vi "Intensity_png.vi"(3 "No of Contours":i32=20, 4 "Job Directory":path=path "/Lacie_20/paulhayden/Documents/EnFlo bits/EnFlo Tun Vel profiles/View_LDA data.tpt", 5 "Intensity Graph":dbl[][](graph)) -> ()   [LabVIEW 2015]
uses:
  Results_plotter_Global.vi
panel:
  out "Folders":string[](array[string])
  out "String":string
  in  "Added labels":i32[](listbox)
  in  "Z Min":dbl=0.97
  in  "Z Max":dbl=1.07
  in  "Save Automatically?":bool
  in  "Auto scale Intensity":bool=TRUE
  in  "Colour":bool=TRUE
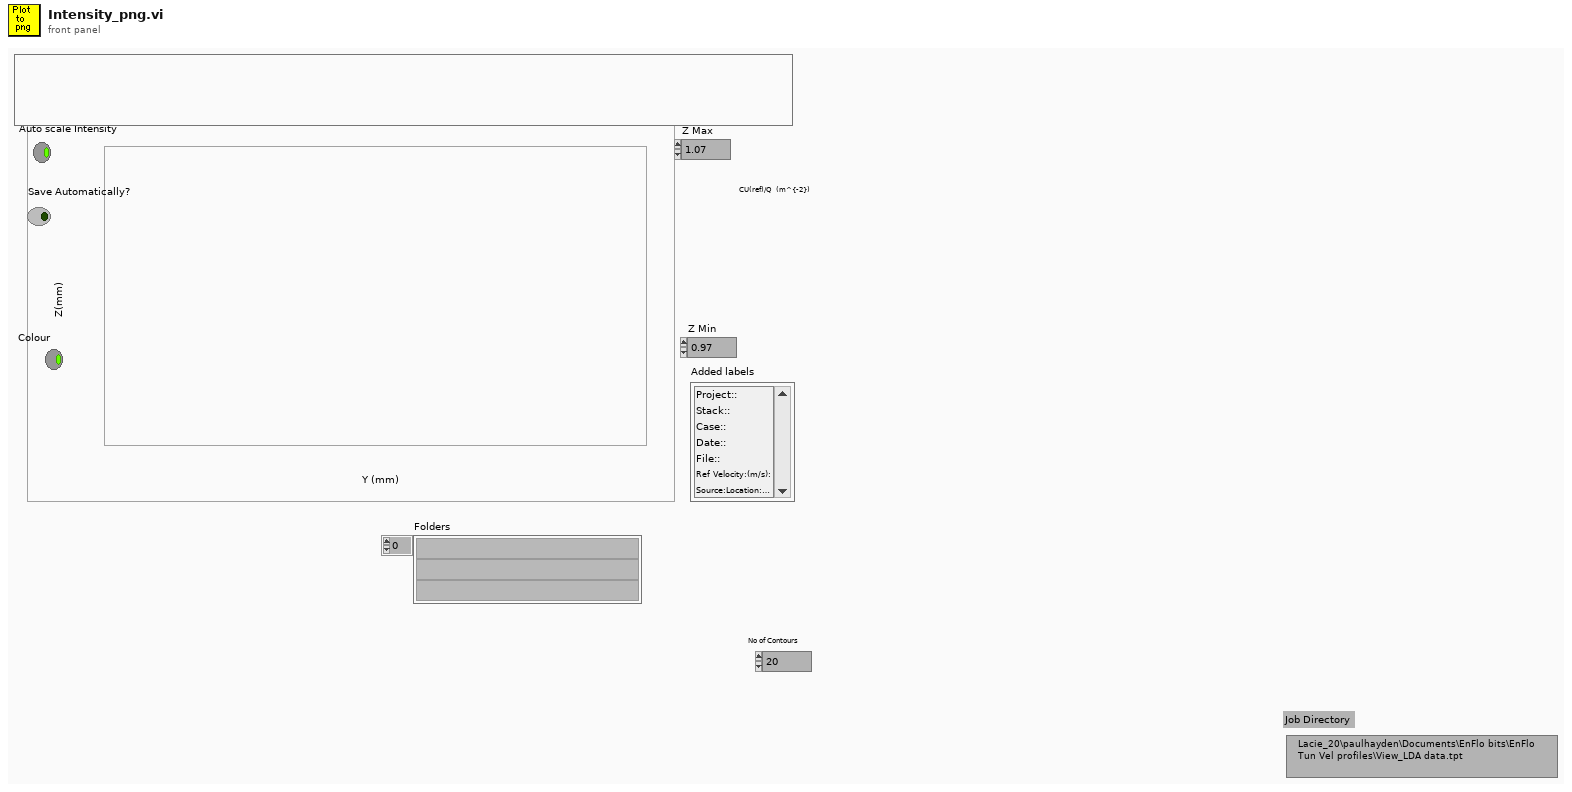
[diagram p1: front panel]
types:
  T1 = typedef "LVRectTypeDef.ctl" = cluster{"left":i16, "top":i16, "right":i16, "bottom":i16}
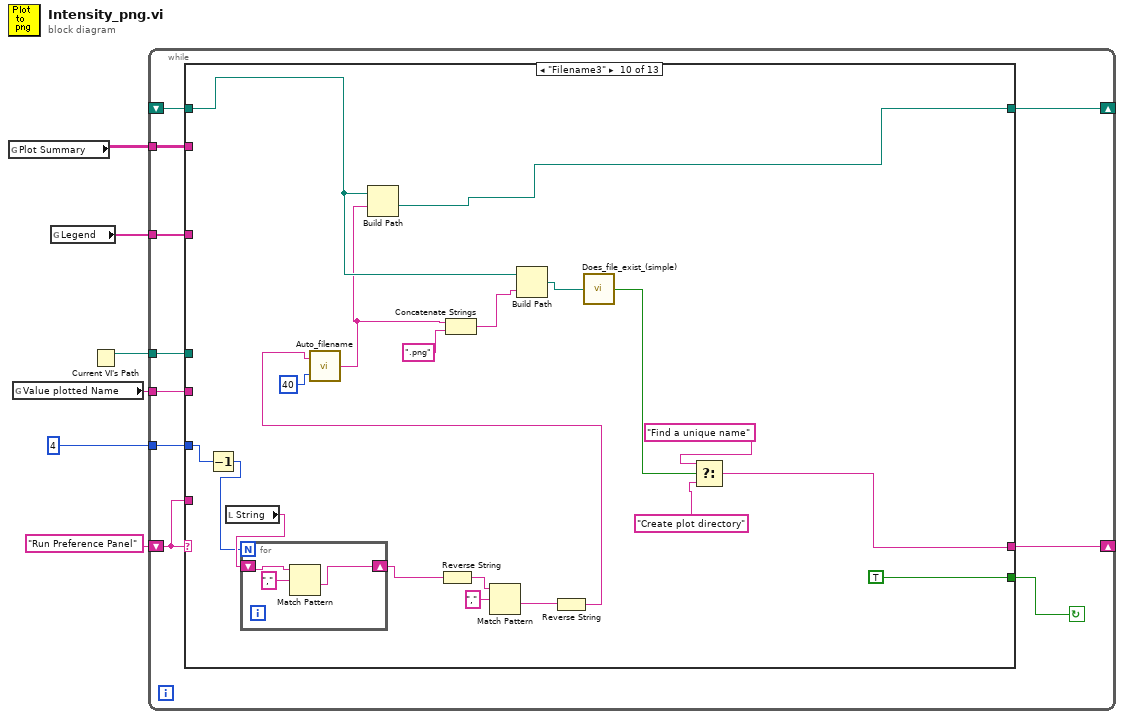
[diagram p0: block diagram]
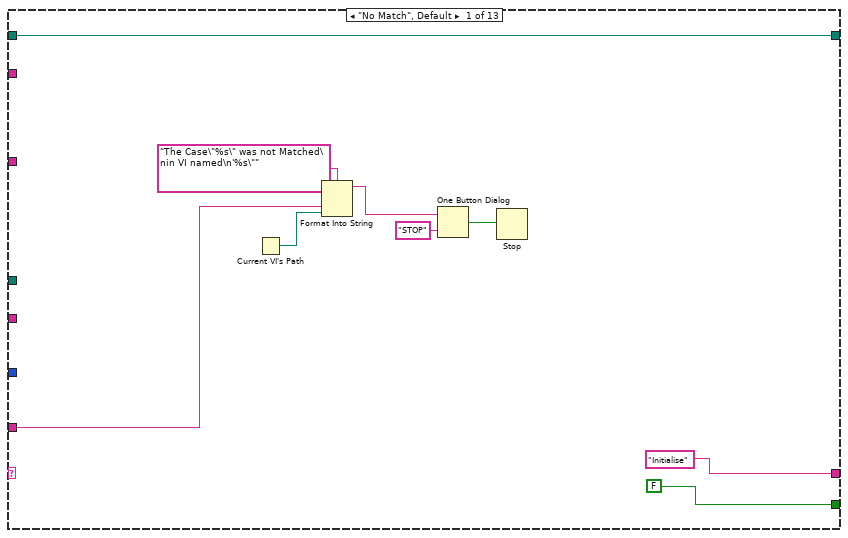
[diagram p2: hidden frame]
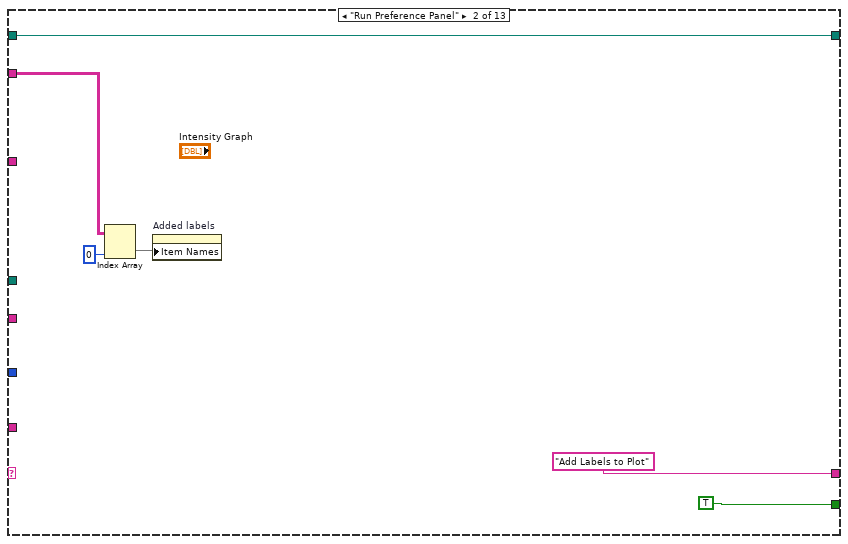
[diagram p3: hidden frame]
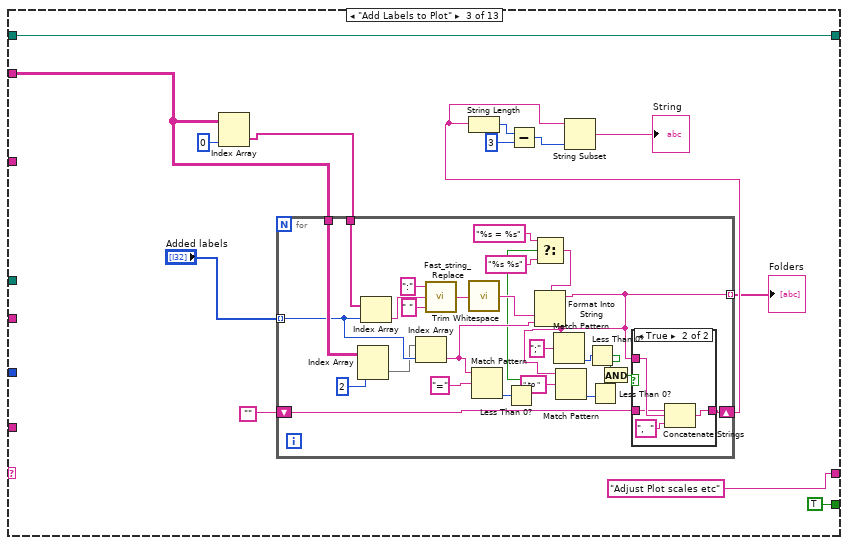
[diagram p4: hidden frame]
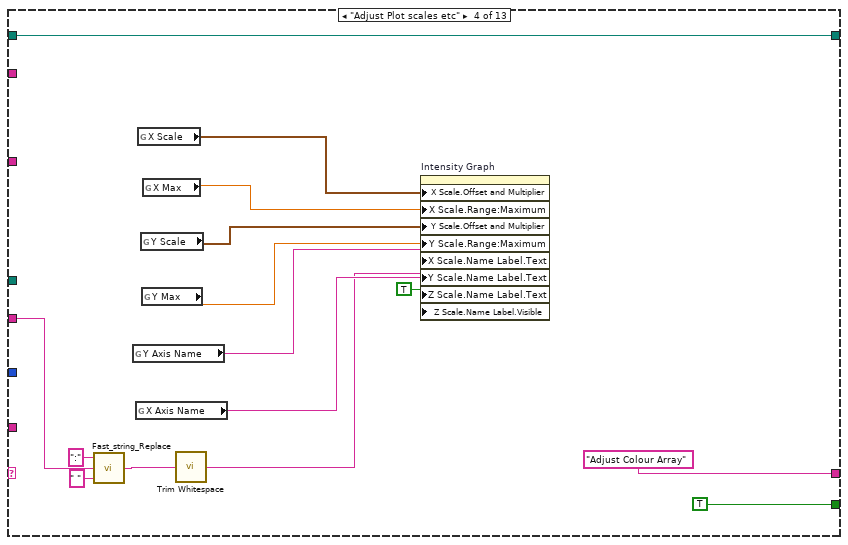
[diagram p6: hidden frame]
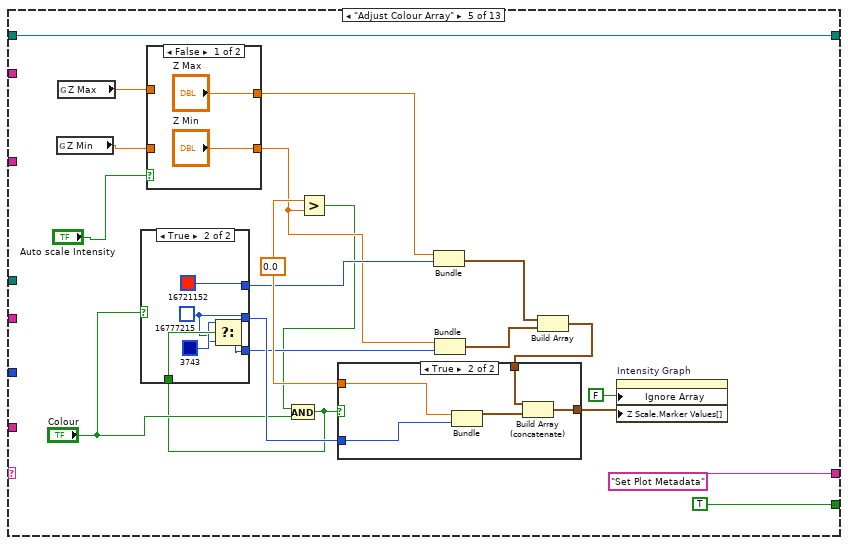
[diagram p7: hidden frame]
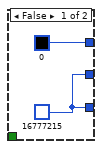
[diagram p8: hidden frame]
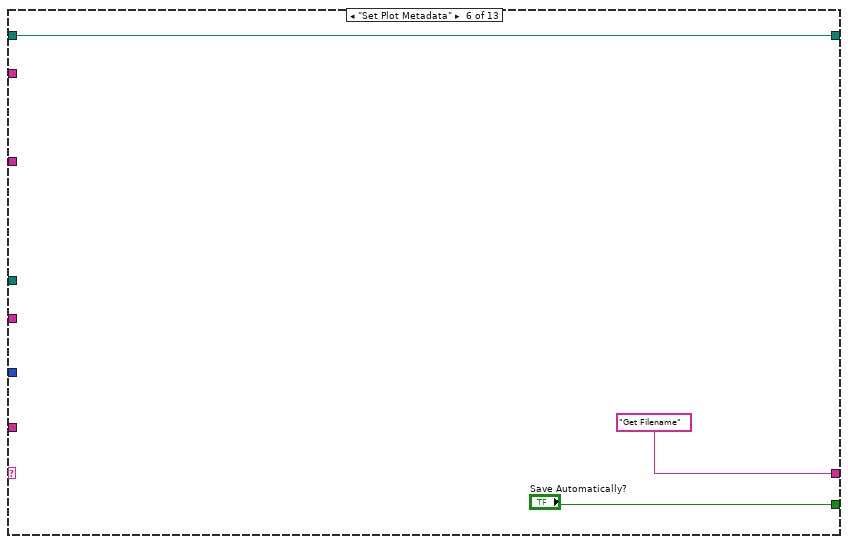
[diagram p11: hidden frame]
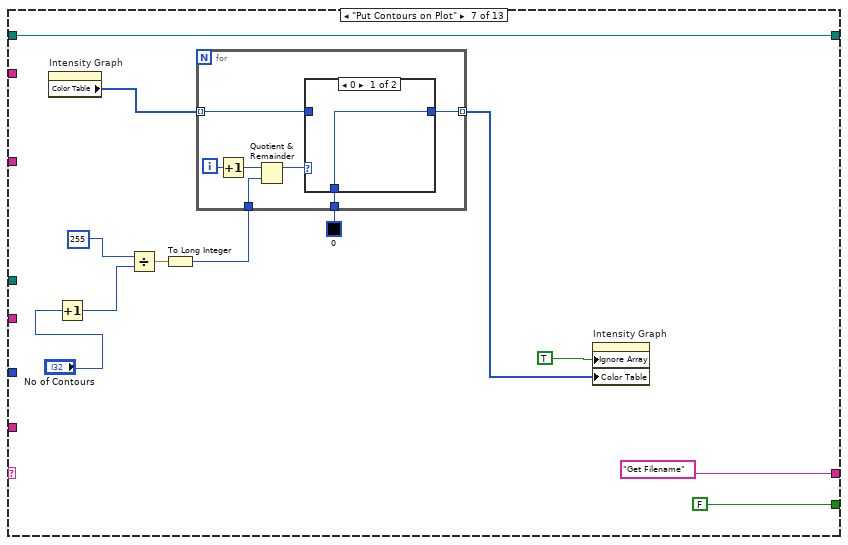
[diagram p12: hidden frame]
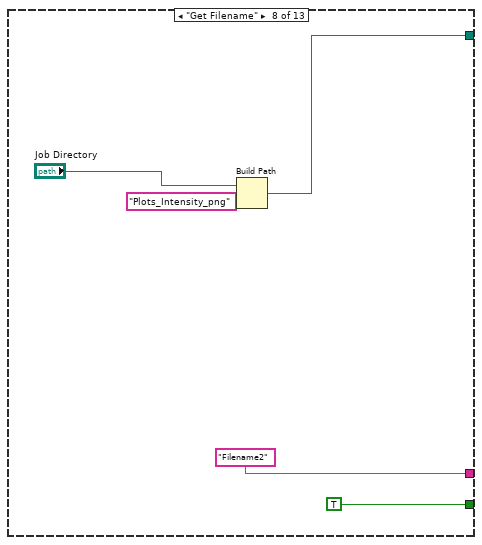
[diagram p14: hidden frame]
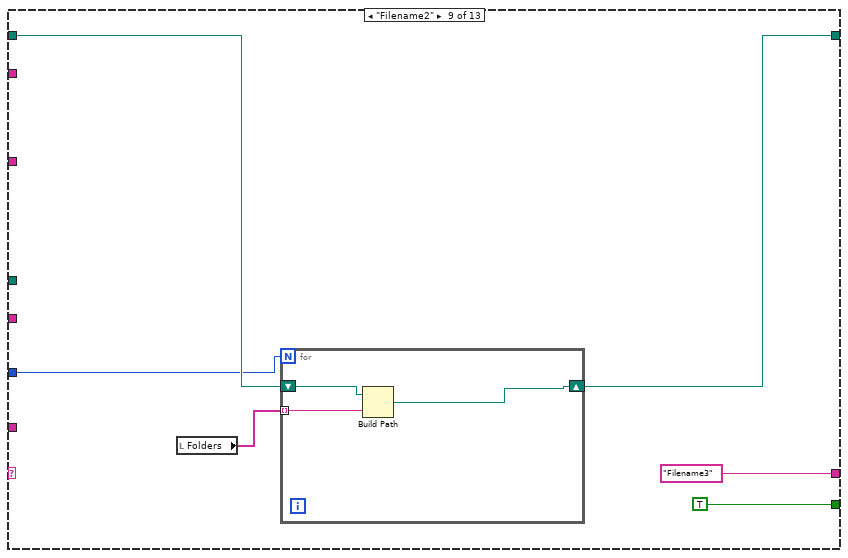
[diagram p15: hidden frame]
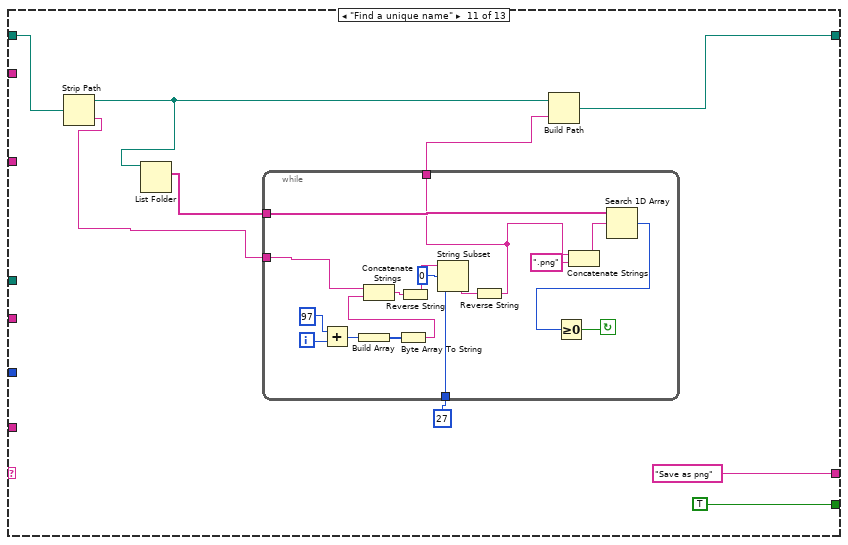
[diagram p16: hidden frame]
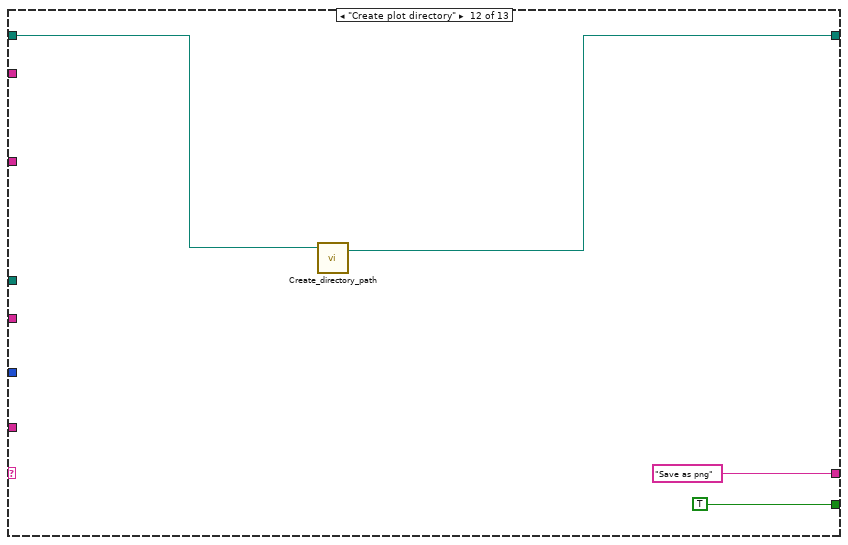
[diagram p17: hidden frame]
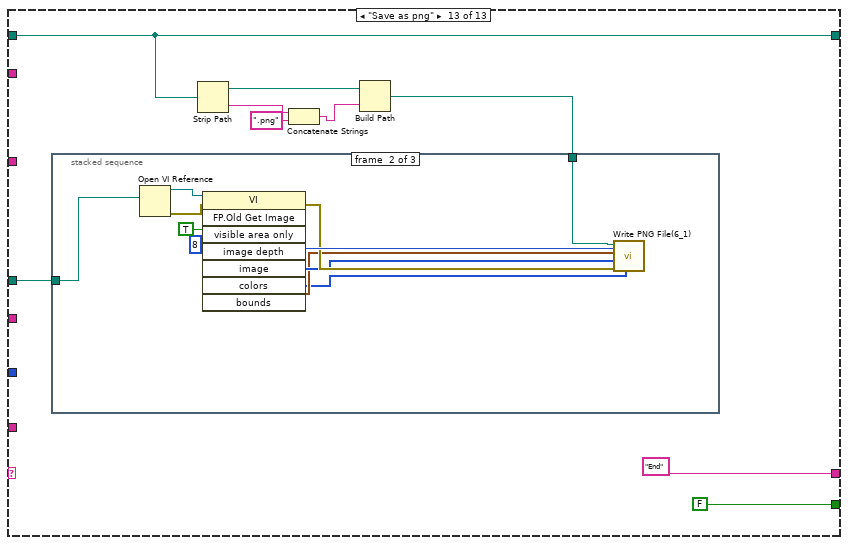
[diagram p18: hidden frame]
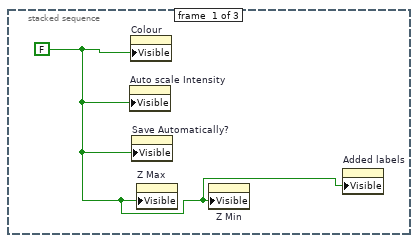
[diagram p19: hidden frame]
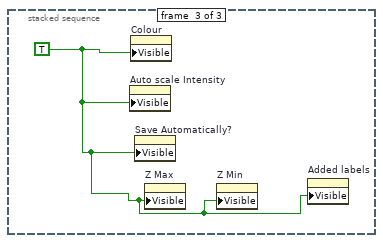
[diagram p20: hidden frame]
diagram:
  n1 = global read "Results_plotter_Global.vi" "Plot Summary"() -> (w2:string[][])
  n2 = global read "Results_plotter_Global.vi" "Value plotted Name"() -> (w4:string)
  n3 = global read "Results_plotter_Global.vi" "Legend"() -> (w3:string[])
  n4 = Current VI's Path() -> (path=w5:path)
  n5 = while {
    shift-left: "Run Preference Panel" -> [w14]
    shift-right: [w15] -> _
    tunnel: w5 -> [w13]
    shift-right: [w12] -> _
    shift-left: _ -> [w11]
    tunnel: w4 -> [w10]
    tunnel: w3 -> [w9]
    tunnel: w2 -> [w8]
    tunnel: 4 -> [w7]
    stop <- w16 continue-if-true
    n6 = case shown="\"Filename3\"" w14 {
      tunnel: [FALSE TRUE TRUE ("Top Level") TRUE ("Top Level") TRUE ("Top Level") "Save Automatically?" FALSE ("Top Level") TRUE ("Top Level") TRUE ("Top Level") TRUE ("Top Level") TRUE ("Top Level") TRUE ("Top Level") FALSE ("Top Level")] -> w16
      tunnel: ["Initialise" "Add Labels to Plot" "Adjust Plot scales etc" "Adjust Colour Array" "Set Plot Metadata" "Get Filename" "Get Filename" "Filename2" "Filename3" w184 "Save as png" "Save as png" "End"] -> w15
      tunnel: w14 -> [w20 _ _ _ _ _ _ _ _ _ _ _ _]
      tunnel: w13 -> [_ _ _ _ _ _ _ _ _ _ _ _ w228]
      tunnel: [w17 w29 w41 w83 w101 w131 w133 w156 w160 w185 w193 w217 w225] -> w12
      tunnel: w11 -> [w17 w29 w41 w83 w101 w131 w133 _ w162 w186 w194 w218 w225]
      tunnel: w10 -> [_ _ _ w82 _ _ _ _ _ _ _ _ _]
      tunnel: w9 -> [_ _ _ _ _ _ _ _ _ _ _ _ _]
      tunnel: w8 -> [_ w27 w45 _ _ _ _ _ _ _ _ _ _]
      tunnel: w7 -> [_ _ _ _ _ _ _ _ w159 w169 _ _ _]
      frame "No Match", Default {
        n7 = Current VI's Path() -> (path=w19:path)
        n8 = Format Into String(format string="The Case\"%s\" was not Matched\nin VI named\n'%s\"" ("Format String"), w20, w19) -> (resulting string=w23:string)  [unwired: 2 in, 1 out]
        n9 = One Button Dialog(message=w23, button name ("OK")="STOP") -> (true=w21:bool)
        n10 = Stop(stop? (T)=w21) -> ()
      }
      frame "Run Preference Panel" {
        n11 = Index Array(array=w27, index (col)=0 ("disabled index (col)")) -> (element=w26:string[])  [unwired: 1 in]
        n12 = property on="Added labels" class="LstBox (strict)"("Item Names"=w26) -> ()  [unwired: 2 in, 2 out]
      }
      frame "Add Labels to Plot" {
        n13 = Index Array(array=w45, index (col)=0 ("disabled index (col)")) -> (element=w43:string[])  [unwired: 1 in]
        n14 = for {
          tunnel: "Added labels" -> [w70] mode=indexing
          tunnel: w43 -> [w72]
          tunnel: w45 -> [w71]
          shift-right: [w61] -> w34
          shift-left: "" -> [w62]
          tunnel: [w46] -> w32 mode=indexing
          n15 = Index Array(array=w71, index (col)=2 ("disabled index (col)")) -> (element=w69:string[])  [unwired: 1 in]
          n16 = Index Array(array=w72, index=w70) -> (element=w66:string)
          n17 = Index Array(array=w69, index=w70) -> (element=w60:string)
          n18 = call "Fast_string_Replace.vi"("Replace match with:"=" ", "Input String"=w66, "regular expression"=":") -> ("Output String"=w65:string)  [unwired: 2 out]
          n19 = call <vilib>:"Trim Whitespace.vi"("string"=w65) -> ("trimmed string"=w64:string)  [unwired: 1 in]
          n20 = Match Pattern(string=w60, regular expression="=") -> (offset past match=w58:i32)  [unwired: 4 out]
          n21 = Less Than 0?(x=w58) -> (x < 0?=w57:bool)
          n22 = Select(t="%s = %s" ("format string"), s=w57, f="%s %s" ("format string")) -> (s? t:f=w54:string)
          n23 = Format Into String(format string=w54, w64, w60) -> (resulting string=w46:string)  [unwired: 2 in, 1 out]
          n24 = Match Pattern(string=w46, regular expression=";") -> (offset past match=w52:i32)  [unwired: 4 out]
          n25 = Match Pattern(string=w46, regular expression=" to ") -> (offset past match=w51:i32)  [unwired: 4 out]
          n26 = Less Than 0?(x=w52) -> (x < 0?=w49:bool)
          n27 = Less Than 0?(x=w51) -> (x < 0?=w50:bool)
          n28 = And(x=w49, y=w50) -> (x .and. y?=w48:bool)
          n29 = case shown="True" w48 {
            tunnel: w62 -> [w73 w75]
            tunnel: [w73 w76] -> w61
            tunnel: w46 -> [_ w77]
            frame False {
            }
            frame True {
              n30 = Concatenate Strings(w75, w77, ",  " ("string")) -> (w76:string)
            }
          }
        }
        "Folders" <- w32
        n31 = String Length(string=w34) -> (length=w37:i32)
        n32 = Subtract(x=w37, y=3) -> (x-y=w35:i32)
        n33 = String Subset(string=w34, length (rest)=w35) -> (substring=→"String":string)  [unwired: 1 in]
      }
      frame "Adjust Plot scales etc" {
        n34 = call "Fast_string_Replace.vi"("Replace match with:"=" ", "Input String"=w82, "regular expression"=":") -> ("Output String"=w79:string)  [unwired: 1 in, 1 out]
        n35 = global read "Results_plotter_Global.vi" "Y Axis Name"() -> (w86:string)
        n36 = global read "Results_plotter_Global.vi" "X Axis Name"() -> (w85:string)
        n37 = global read "Results_plotter_Global.vi" "X Scale"() -> (w91:cluster{"Xo":dbl, "delta X":dbl})
        n38 = global read "Results_plotter_Global.vi" "Y Scale"() -> (w89:cluster{"Xo":dbl, "delta X":dbl})
        n39 = global read "Results_plotter_Global.vi" "Y Max"() -> (w88:dbl)
        n40 = global read "Results_plotter_Global.vi" "X Max"() -> (w90:dbl)
        n41 = call <vilib>:"Trim Whitespace.vi"("string"=w79) -> ("trimmed string"=w78:string)  [unwired: 1 in]
        n42 = property on="Intensity Graph" class="IntGraph (strict)"("X Scale.Offset and Multiplier"=w91, "X Scale.Range:Maximum"=w90, "Y Scale.Offset and Multiplier"=w89, "Y Scale.Range:Maximum"=w88, "X Scale.Name Label.Text"=w86, "Y Scale.Name Label.Text"=w85, "Z Scale.Name Label.Text"=w78, "Z Scale.Name Label.Visible"=TRUE) -> ()  [unwired: 2 in, 2 out]
      }
      frame "Adjust Colour Array" {
        w112 = 0.0 ("max Z value")
        n43 = global read "Results_plotter_Global.vi" "Z Min"() -> (w97:dbl)
        n44 = global read "Results_plotter_Global.vi" "Z Max"() -> (w99:dbl)
        n45 = case shown="False" "Auto scale Intensity" {
          tunnel: ["Z Max" w123] -> w100
          tunnel: w99 -> [_ w123]
          tunnel: ["Z Min" w122] -> w98
          tunnel: w97 -> [_ w122]
          frame False {
          }
          frame True {
          }
        }
        n46 = Greater?(x=w112, y=w98) -> (0:w95:bool)
        n47 = And(x=w95, y="Colour") -> (x .and. y?=w93:bool)
        n48 = case shown="True" "Colour" {
          tunnel: [w114 w115] -> w108
          tunnel: [u32 0 u32 16721152] -> w107
          tunnel: [w114 w116] -> w103
          tunnel: w93 -> [_ w118]
          frame False {
            w114 = u32 16777215
          }
          frame True {
            w115 = u32 16777215
            n49 = Select(t=u32 3743, s=w118, f=w115) -> (s? t:f=w116:u32)
          }
        }
        n50 = Bundle("Z Max"=w100, w107) -> (w109:cluster{"Z Max":dbl, u32})  [unwired: 1 in]
        n51 = Bundle("Z Min"=w98, w103) -> (w111:cluster{"Z Min":dbl, u32})  [unwired: 1 in]
        n52 = Build Array(w109, w111) -> (w110:cluster{"Z Min":dbl, u32}[])
        n53 = case shown="True" w93 {
          tunnel: w110 -> [w124 w129]
          tunnel: [w124 w127] -> w105
          tunnel: w108 -> [_ w126]
          tunnel: w112 -> [_ w125]
          frame False {
          }
          frame True {
            n54 = Bundle("max Z value"=w125, w126) -> (w128:cluster{"max Z value":dbl, u32})  [unwired: 1 in]
            n55 = Build Array (concatenate)(w129, w128) -> (w127:cluster{"max Z value":dbl, u32}[])
          }
        }
        n56 = property on="Intensity Graph" class="IntGraph (strict)"("Ignore Array"=FALSE, "Z Scale.Marker Values[]"=w105) -> ()  [unwired: 2 in, 2 out]
      }
      frame "Set Plot Metadata" {
      }
      frame "Put Contours on Plot" {
        n57 = property on="Intensity Graph" class="IntGraph (strict)"() -> ("Color Table"=w136:u32[])  [unwired: 2 in, 2 out]
        n58 = Increment(x="No of Contours") -> (x+1=w141:i32)
        n59 = Divide(x=255, y=w141) -> (x/y=w140:dbl)
        n60 = To Long Integer(number=w140) -> (32bit integer=w138:i32)
        n61 = for {
          tunnel: w138 -> [w150]
          tunnel: [w147] -> w135 mode=indexing
          tunnel: w136 -> [w146] mode=indexing
          tunnel: u32 0 -> [w145]
          i -> [w151]
          n62 = Increment(x=w151) -> (x+1=w148:i32)
          n63 = Quotient & Remainder(x=w148, y=w150) -> (x-y*floor(x/y)=w149:i32)  [unwired: 1 out]
          n64 = case shown="0" w149 {
            tunnel: [w152 w153] -> w147
            tunnel: w146 -> [_ w153]
            tunnel: w145 -> [w152 _]
            frame 0 {
            }
            frame 1, Default {
            }
          }
        }
        n65 = property on="Intensity Graph" class="IntGraph (strict)"("Ignore Array"=TRUE, "Color Table"=w135) -> ()  [unwired: 2 in, 2 out]
      }
      frame "Get Filename" {
        n66 = Build Path(base path="Job Directory", name or relative path="Plots_Intensity_png") -> (appended path=w156:path)
      }
      frame "Filename2" {
        n67 = local read "Folders"() -> (w161:string[])
        n68 = for {
          N: w159 -> [_]
          shift-right: [w165] -> w160
          shift-left: w162 -> [w167]
          tunnel: w161 -> [w166] mode=indexing
          n69 = Build Path(base path=w167, name or relative path=w166) -> (appended path=w165:path)
        }
      }
      frame "Filename3" {
        n70 = Decrement(x=w169) -> (x-1=w168:i32)
        n71 = local read "String"() -> (w171:string)
        n72 = for {
          N: w168 -> [_]
          shift-right: [w188] -> w170
          shift-left: w171 -> [w189]
          n73 = Match Pattern(string=w189, regular expression=",") -> (after substring=w188:string)  [unwired: 1 in, 3 out]
        }
        n74 = Reverse String(1:w170) -> (0:w174:string)
        n75 = Match Pattern(string=w174, regular expression=",") -> (after substring=w173:string)  [unwired: 1 in, 3 out]
        n76 = Reverse String(1:w173) -> (0:w172:string)
        n77 = call "Auto_filename.vi"("Filename Max length"=40, "Prefix"=w172) -> ("Filename"=w177:string)
        n78 = Build Path(base path=w186, name or relative path=w177) -> (appended path=w185:path)
        n79 = Concatenate Strings(w177, ".png" ("string")) -> (w182:string)
        n80 = Build Path(base path=w186, name or relative path=w182) -> (appended path=w181:path)
        n81 = call "Does_file_exist_(simple).vi"("Pathname"=w181) -> ("exists?"=w180:bool)
        n82 = Select(t="Find a unique name", s=w180, f="Create plot directory") -> (s? t:f=w184:string)
      }
      frame "Find a unique name" {
        n83 = Strip Path(path=w194) -> (stripped path=w192:path, name=w196:string)
        n84 = List Folder(path=w192) -> (filenames=w191:string[])  [unwired: 3 in, 3 out]
        n85 = while {
          tunnel: w196 -> [w216]
          tunnel: 27 ("Max Length") -> [w215]
          tunnel: [w201] -> w197
          tunnel: w191 -> [w205]
          i -> [w206]
          stop <- w203 continue-if-true
          n86 = Add(x=97, y=w206) -> (x+y=w213:i32)
          n87 = Build Array(w213) -> (w214:i32[])
          n88 = Byte Array To String(unsigned byte array=w214) -> (string=w211:string)
          n89 = Concatenate Strings(w216, w211) -> (w209:string)
          n90 = Reverse String(1:w209) -> (0:w210:string)
          n91 = String Subset(string=w210, offset (0)=0, length (rest)=w215) -> (substring=w208:string)
          n92 = Reverse String(1:w208) -> (0:w201:string)
          n93 = Concatenate Strings(w201, ".png" ("string")) -> (w200:string)
          n94 = Search 1D Array(1D array=w205, element=w200) -> (index of element=w204:i32)  [unwired: 1 in]
          n95 = Greater Or Equal To 0?(x=w204) -> (x >= 0?=w203:bool)
        }
        n96 = Build Path(base path=w192, name or relative path=w197) -> (appended path=w193:path)
      }
      frame "Create plot directory" {
        n97 = call "Create_directory_path.vi"("Path name"=w218) -> ("Path name Out"=w217:path)  [unwired: 2 in, 1 out]
      }
      frame "Save as png" {
        n98 = Strip Path(path=w225) -> (stripped path=w226:path, name=w224:string)
        n99 = Concatenate Strings(w224, ".png" ("string")) -> (w223:string)
        n100 = Build Path(base path=w226, name or relative path=w223) -> (appended path=w221:path)
        n101 = stacked-sequence {
          tunnel: w228 -> [_ w238 _]
          tunnel: w221 -> [_ w231 _]
          frame #0 {
            w230 = FALSE ("Visible")
            n102 = property on="Auto scale Intensity" class="Bool (strict)"("Visible"=w230) -> ()  [unwired: 2 in, 2 out]
            n103 = property on="Colour" class="Bool (strict)"("Visible"=w230) -> ()  [unwired: 2 in, 2 out]
            n104 = property on="Save Automatically?" class="Bool (strict)"("Visible"=w230) -> ()  [unwired: 2 in, 2 out]
            n105 = property on="Z Max" class="DigNum (strict)"("Visible"=w230) -> ()  [unwired: 2 in, 2 out]
            n106 = property on="Z Min" class="DigNum (strict)"("Visible"=w230) -> ()  [unwired: 2 in, 2 out]
            n107 = property on="Added labels" class="LstBox (strict)"("Visible"=w230) -> ()  [unwired: 2 in, 2 out]
          }
          frame #1 {
            w236 = 8 ("image depth")
            n108 = Open VI Reference(vi path=w238) -> (vi reference=w240:refnum<vi>, error out=w239:errorcluster)  [unwired: 5 in]
            n109 = invoke class="VI" method="FP.Old Get Image"(reference=w240, error in=w239, "visible area only"=TRUE, "image depth"=w236) -> (error out=w235:errorcluster, "image"=w234:u8[], "colors"=w232:u32[], "bounds"=w233:T1)  [unwired: 4 in, 4 out]
            n110 = call <vilib>:"Write PNG File(6_1).vi"("color table"=w232, "depth"=w236, "error in (no error)"=w235, "flattened image data"=w234, "rect"=w233, "path to PNG file"=w231) -> ()  [unwired: 4 in, 2 out]
          }
          frame #2 {
            w241 = TRUE ("Visible")
            n111 = property on="Auto scale Intensity" class="Bool (strict)"("Visible"=w241) -> ()  [unwired: 2 in, 2 out]
            n112 = property on="Colour" class="Bool (strict)"("Visible"=w241) -> ()  [unwired: 2 in, 2 out]
            n113 = property on="Save Automatically?" class="Bool (strict)"("Visible"=w241) -> ()  [unwired: 2 in, 2 out]
            n114 = property on="Z Max" class="DigNum (strict)"("Visible"=w241) -> ()  [unwired: 2 in, 2 out]
            n115 = property on="Z Min" class="DigNum (strict)"("Visible"=w241) -> ()  [unwired: 2 in, 2 out]
            n116 = property on="Added labels" class="LstBox (strict)"("Visible"=w241) -> ()  [unwired: 2 in, 2 out]
          }
        }
      }
    }
  }
